vi "LSX Send String.vi"(0 "lLSID":i32, 1 "bReadLine":i32, 5 "pcStr":string, 7 "pcRet":string, 9 "lMaxLen":i32, 11 "error in (no error)":errorcluster, 12 "lTimeOut":i32) -> (4 "function return":i32, 6 "pcStr out":string, 8 "pcRet out":string, 15 "error out":errorcluster)   [LabVIEW 2018, in "Tango.lvlib"]
doc: "TANGOAPI int TANGOCALL LSX_SendString (int lLSID, char *pcStr, char *pcRet, int lMaxLen, BOOL bReadLine, int lTimeOut);"
uses:
  <userlib>/Tango/Tango.lvlib
  <userlib>/Tango/Tango_DLL.dll
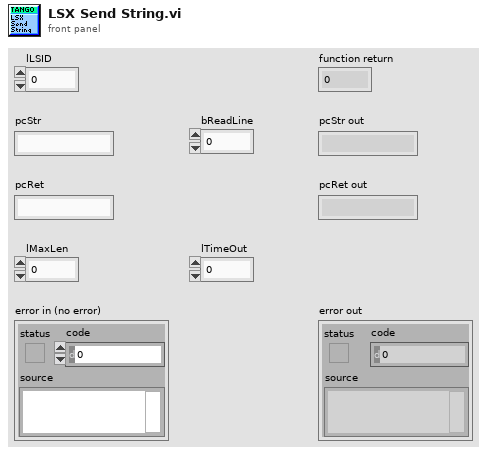
[diagram p1: front panel]
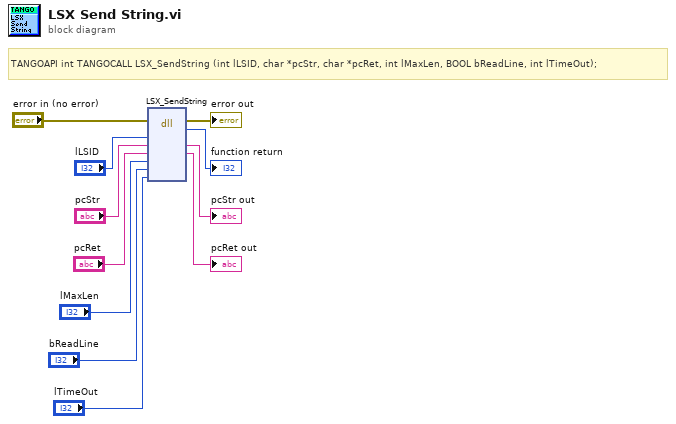
[diagram p0: block diagram]
diagram:
  # "TANGOAPI int TANGOCALL LSX_SendString (int lLSID, char *pcStr, char *pcRet, int lMaxLen, BOOL bReadLine, int lTimeOut);"
  n1 = dll-call lib="C:/Program Files (x86)/National Instruments/LabVIEW 2018/user.lib/Tango/Tango_DLL.*" fn="LSX_SendString"(error in="error in (no error)", "lLSID"="lLSID", "pcStr"="pcStr", "pcRet"="pcRet", "lMaxLen"="lMaxLen", "bReadLine"="bReadLine", "lTimeOut"="lTimeOut") -> (error out=→"error out":errorcluster, →"function return":i32, "pcStr"=→"pcStr out":string, "pcRet"=→"pcRet out":string)  [unwired: 6 in, 1 out]
